vi "TurnOFF_ON (SubVI).vi"(8 "error constant":errorcluster, 9 "TurnOFF/ON":string(combo)="TurnOFF", 10 "DAQmx Device Name":tag, 11 "VISA":refnum<visa-resource-name>) -> (0 "error constant 2":errorcluster)   [LabVIEW 2017]
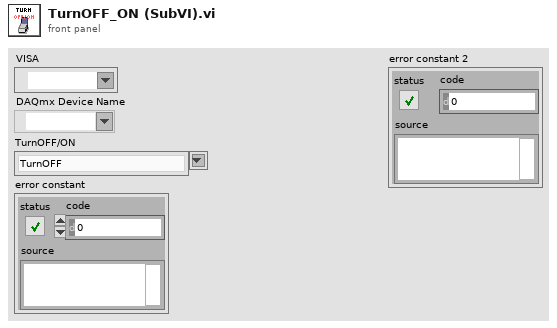
[diagram p1: front panel]
types:
  T1 = enum16{"DB0", "DB1", "DB2", "DB3", "DB4", "DB5", "DB6", "DB7", "DB8", "DB9", "DB10", "DB11", "A0", "A1", "RW", "LDAC", "ADMAIN1", "ADMAIN2", "ADMAIN3", "G1", "CS", "CLR", "P0", "P1"}
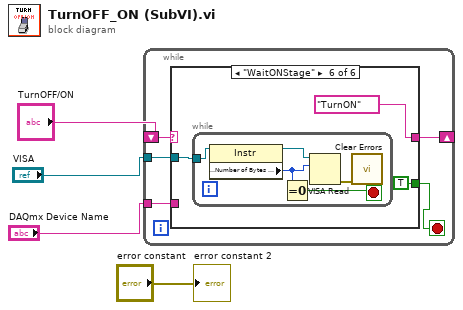
[diagram p0: block diagram]
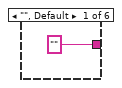
[diagram p2: hidden frame]
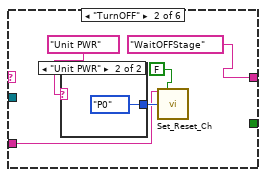
[diagram p3: hidden frame]
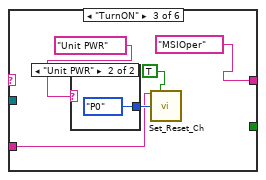
[diagram p5: hidden frame]
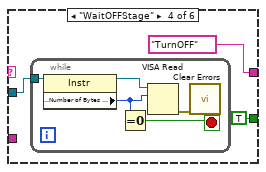
[diagram p7: hidden frame]
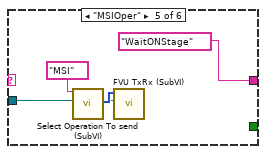
[diagram p8: hidden frame]
diagram:
  n1 = while {
    tunnel: "DAQmx Device Name" -> [w8]
    shift-right: [w7] -> _
    shift-left: "TurnOFF/ON" -> [w9]
    tunnel: "VISA" -> [w5]
    stop <- w6 stop-if-true
    n2 = case shown="\"WaitONStage\"" w9 {
      tunnel: w8 -> [_ w12 w18 _ _ _]
      tunnel: ["" ("Combo Box") "WaitOFFStage" ("Combo Box") "MSIOper" ("Combo Box") "TurnOFF" ("Combo Box") "WaitONStage" ("Combo Box") "TurnON" ("Combo Box")] -> w7
      tunnel: [_ _ _ TRUE _ TRUE] -> w6
      tunnel: w5 -> [_ _ _ w24 w31 w36]
      frame "", Default {
      }
      frame "TurnOFF" {
        n3 = case shown="\"Unit PWR\"" "Unit PWR" ("Combo Box") {
          tunnel: [_ T1."P0" ("Ch 2")] -> w15
          frame "False", Default {
          }
          frame "Unit PWR" {
          }
        }
        n4 = call "Set_Reset_Ch.vi"("device name"=w12, "SetReset"=FALSE ("ON(T)/OFF(F)"), "Ch"=w15) -> ()  [unwired: 12 in, 1 out]
      }
      frame "TurnON" {
        n5 = case shown="\"Unit PWR\"" "Unit PWR" ("Combo Box") {
          tunnel: [_ T1."P0" ("Ch 2")] -> w21
          frame "False", Default {
          }
          frame "Unit PWR" {
          }
        }
        n6 = call "Set_Reset_Ch.vi"("device name"=w18, "SetReset"=TRUE ("ON(T)/OFF(F)"), "Ch"=w21) -> ()  [unwired: 12 in, 1 out]
      }
      frame "WaitOFFStage" {
        n7 = while {
          tunnel: w24 -> [w27]
          stop <- w26 stop-if-true
          n8 = property class="Instr"(reference=w27) -> (reference out=w30:refnum<visa-resource-name>, "Serial Settings:Number of Bytes at Serial Port"=w28:u32)  [unwired: 1 in, 1 out]
          n9 = Equal To 0?(x=w28) -> (x = 0?=w26:bool)
          n10 = VISA Read(VISA resource name=w30, byte count=w28) -> (error out=w29:errorcluster)  [unwired: 1 in, 3 out]
          n11 = call <vilib>:"Clear Errors.vi"("error in (no error)"=w29) -> ()  [unwired: 5 in, 2 out]
        }
      }
      frame "MSIOper" {
        n12 = call "Select Operation To send (SubVI).vi"("Combo Box"="MSI") -> ("write"=w32:u8[])  [unwired: 18 in]
        n13 = call "FVU TxRx (SubVI).vi"("VISA in"=w31, "write"=w32) -> ()  [unwired: 6 in, 4 out]
      }
      frame "WaitONStage" {
        n14 = while {
          tunnel: w36 -> [w38]
          stop <- w39 stop-if-true
          n15 = property class="Instr"(reference=w38) -> (reference out=w42:refnum<visa-resource-name>, "Serial Settings:Number of Bytes at Serial Port"=w40:u32)  [unwired: 1 in, 1 out]
          n16 = Equal To 0?(x=w40) -> (x = 0?=w39:bool)
          n17 = VISA Read(VISA resource name=w42, byte count=w40) -> (error out=w41:errorcluster)  [unwired: 1 in, 3 out]
          n18 = call <vilib>:"Clear Errors.vi"("error in (no error)"=w41) -> ()  [unwired: 5 in, 2 out]
        }
      }
    }
  }
  "error constant 2" <- "error constant"
